vi "GUI_TestStand_Screen1.vi"() -> ()   [LabVIEW 2013]
uses:
  Shared/GUI_Template/GUI_master/tcp_new_data_event.ctl
  Shared/GUI_Template/GUI_master/tcp new data cluster.ctl
  Fire button.ctl
panel:
  in  "RepRate::6":dbl=25.5 caption="Rep\nrate" min=0.0 max=0.0 format="%#.2f"
  out "flow::11":dbl=25.5 caption="PR4000 Flow" min=0.0 max=0.0 format="%_4f"
  out "pressure chart":dbl(graph) caption="Baratron pressure"
  in  "MaxCounts::13":dbl=25.5 caption="Max counts TS-ChromexCam" min=0.0 max=1000.0 format="%_4f"
  out "OK Button 4":bool
  in  "MaxCounts::14":dbl=25.5 caption="Max counts TS-InputNearField" min=0.0 max=1000.0 format="%_4f"
  out "OK Button 3":bool
  in  "MaxCounts::12":dbl=25.5 caption="Max counts TS-Mode1" min=0.0 max=999999999.0 format="%_4f"
  out "OK Button 2":bool
  in  "valve::11":bool caption="Valve"
  in  "pressure::11":dbl=25.5 caption="PR4000 Pressure" min=0.0001 max=30.0 format="%_4f"
  in  "BaratronPressure::9":dbl=25.5 caption="Baratron Pressure" min=0.01 max=10.0 format="%_4f"
  in  "GUIdevice 14":string="TS-InputNearField"
  in  "trigger::14":bool caption="TS-InputNearField"
  in  "trigger::13":bool caption="TS-ChromexCam"
  in  "GUIdevice 13":string="TS-ChromexCam"
  in  "trigger::12":bool caption="TS-Mode1"
  in  "GUIdevice 12":string="TS-Mode1"
  in  "trigger::8":bool caption="TS-Periscope"
  in  "GUIdevice 11":string="TS-PR4000"
  in  "fire::6":string="TS-shotcontrol"
  in  "Fire Button":T1
  in  "Mode::6":bool caption="Mode"
  out "transmission chart":dbl(graph) caption="Transmission [%]"
  in  "EnergyIn::10":dbl=25.5 caption="Pulse energy [uJ]" min=-5.0 max=5.0 format="%_3f"
  in  "EnergyTransmission::10":dbl=-1.0 caption="Transmission [%]" min=0.0001 max=30.0 format="%_3f"
  in  "GUIdevice 10":string="TS-Analysis"
  in  "GUIdevice 9":string="GP1teststand"
  out "OK Button":bool
  in  "MaxCounts::8":dbl=25.5 caption="Max counts TS-Periscope" min=0.01 max=10.0 format="%_4f"
  in  "GUIdevice 8":string="TS-Periscope"
  in  "Trigger.Low Level::7":dbl caption="Level" min=-0.1 max=0.1
  in  "Trigger.Mode::7":T2(ring) caption="Mode"
  in  "delay.Channel_A::4":dbl=40.15 caption="Delay A" min=-0.1 max=0.1 format="%^_4g"
  in  "delay.Channel_D::5":dbl=40.15 caption="Delay D" min=-0.1 max=0.1 format="%_4f"
  in  "delay.Channel_C::5":dbl=40.15 caption="Delay C" min=-0.1 max=0.1 format="%^_6e"
  in  "delay.Channel_B::5":dbl=40.15 caption="Delay B" min=-0.1 max=0.1 format="%_4f"
  in  "delay.Channel_A::5":dbl=40.15 caption="Delay A" min=-0.1 max=0.1 format="%^_6e"
  in  "delay.Channel_D::4":dbl=40.15 caption="Delay D" min=-0.1 max=0.1 format="%_4f"
  in  "delay.Channel_C::4":dbl=40.15 caption="Delay C" min=0.1 max=10.0 format="%_4f"
  in  "delay.Channel_B::4":dbl=40.15 caption="Delay B" min=-0.1 max=0.1 format="%_4f"
  in  "Digitizer Traces":T3 {"offset::7" min=0.0 max=5000.0 format="%_4f"; "verticalrange::7" min=0.0 max=500.0 format="%_4f"}
  in  "position::3":dbl=40.15 caption="Arcus 2 stage \nposition" min=-7.5 max=7.5 format="%_4f"
  in  "position::2":dbl=25.5 caption="Arcus 1 stage" min=-25.0 max=25.0 format="%_4f"
  in  "wangle::1":dbl caption="w" min=0.0 max=50.0 format="%_4f"
  in  "vangle::1":dbl caption="v" min=0.0 max=50.0 format="%_4f"
  in  "uangle::1":dbl=0.5 caption="u" min=0.0 max=50.0 format="%_4f"
  in  "ypos::1":dbl caption="y" min=-7.5 max=7.5 format="%_4f"
  in  "zpos::1":dbl caption="z" min=-12.0 max=12.0 format="%_4f"
  in  "xpos::1":dbl=0.5 caption="x" min=-25.0 max=25.0 format="%_4f"
  in  "GUIdevice 7":string="TS-digitizer-1"
  out "error IO 2":errorcluster
  in  "insert tag":bool=TRUE
  out "tcp data event":T4
  in  "GUIdevice 5":string="TS-dg535-2"
  in  "GUIdevice 4":string="TS-dg535-1"
  in  "GUIdevice 6":string="TS-shotcontrol"
  in  "GUIdevice 3":string="TSArcus2"
  in  "GUIdevice 2":string="TSArcus1"
  in  "GUIdevice 1":string="TS-hexapod"
  in  "stop":bool
  in  "UDP error message":string
  # "TEST STAND CONTROL CENTER"
  # "DIGITIZER"
  # "FOCUS LENS"
  # "SHOT CONTROL"
  # "Trigger"
  # "Camera triggers"
  # "Pressures"
  # "CALCULATIONS"
  # "DG 1"
  # "DG 2"
  # "MODE 1"
  # "HEXAPOD"
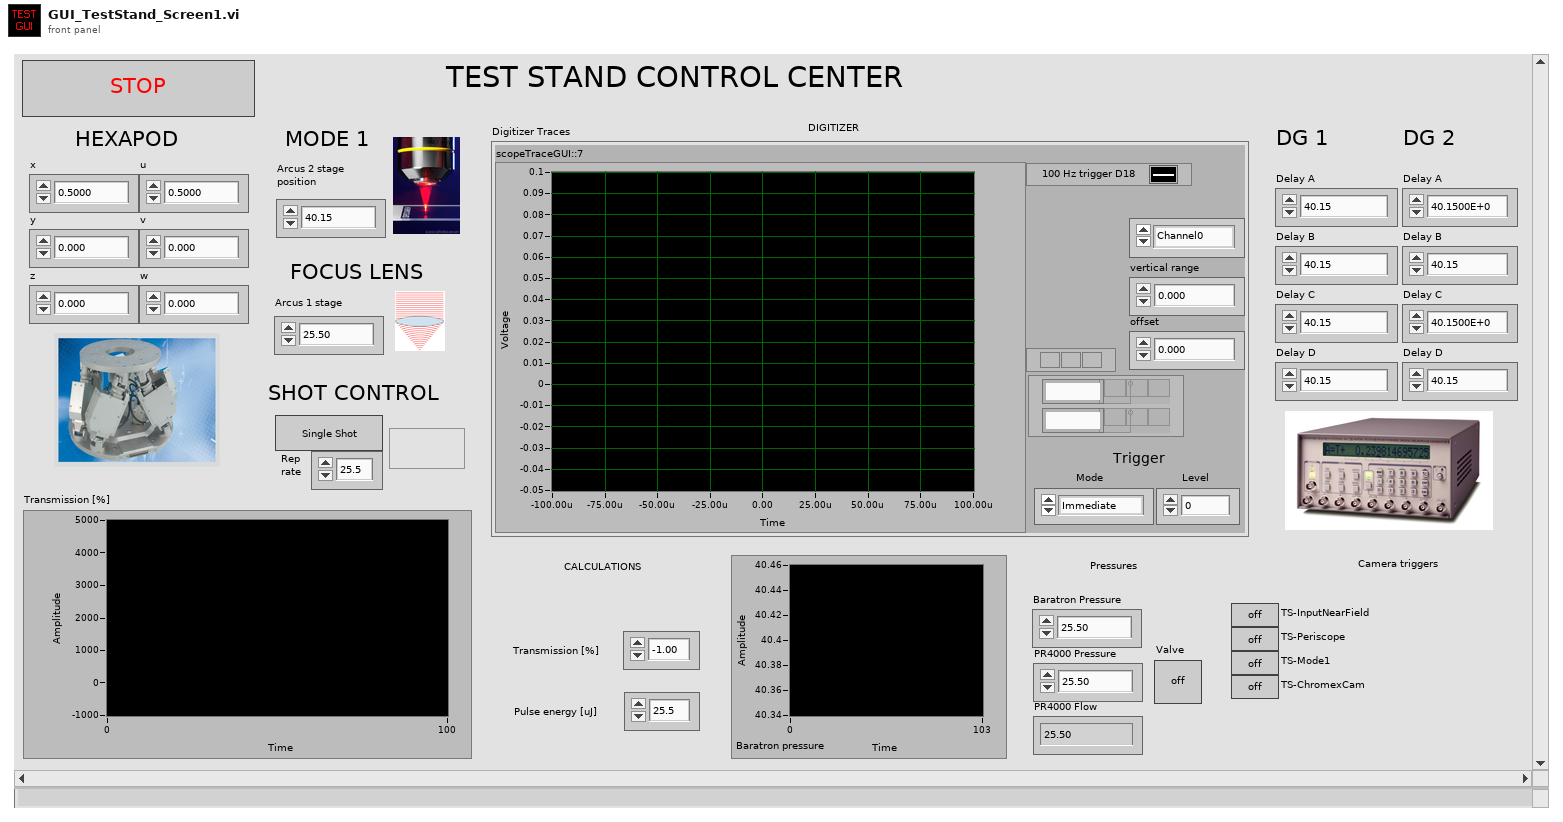
[diagram p1: front panel]
types:
  T1 = typedef "Fire button.ctl" = bool
  T2 = enum16{"Immediate", "Analog Edge", "Analog Window", "Analog Hysteresis", "Video", "Digital Edge"}
  T3 = cluster{"verticalrange::7":dbl, "Channel::7":enum16{"Channel0", "Channel1", "Channel2"}, "scopeTraceGUI::7":waveform(dbl)[], "offset::7":dbl}
  T4 = typedef "tcp_new_data_event.ctl" = refnum<user-event>
  T5 = typedef "tcp new data cluster.ctl" = cluster{"EventEnum":enum16{"new data", "connection status update"}, "Device name":string}
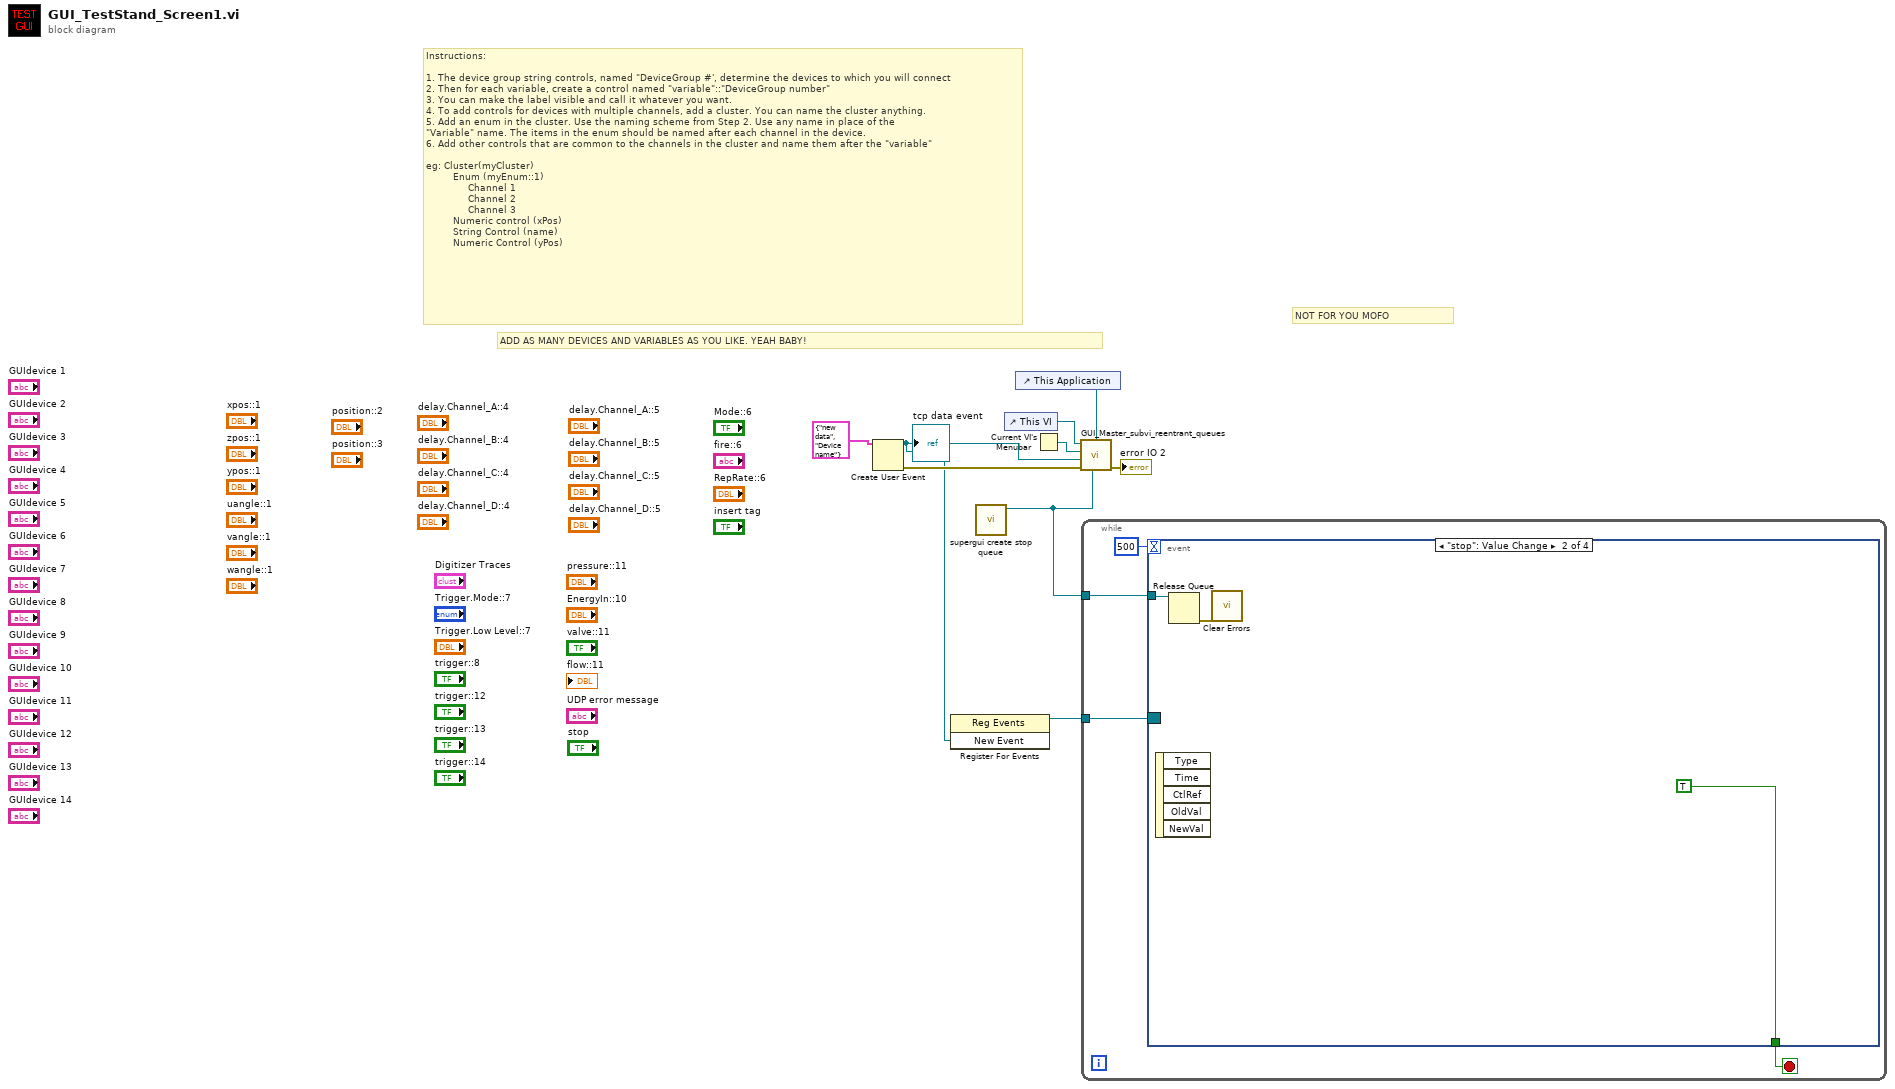
[diagram p0: block diagram]
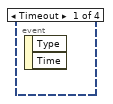
[diagram p2: hidden frame]
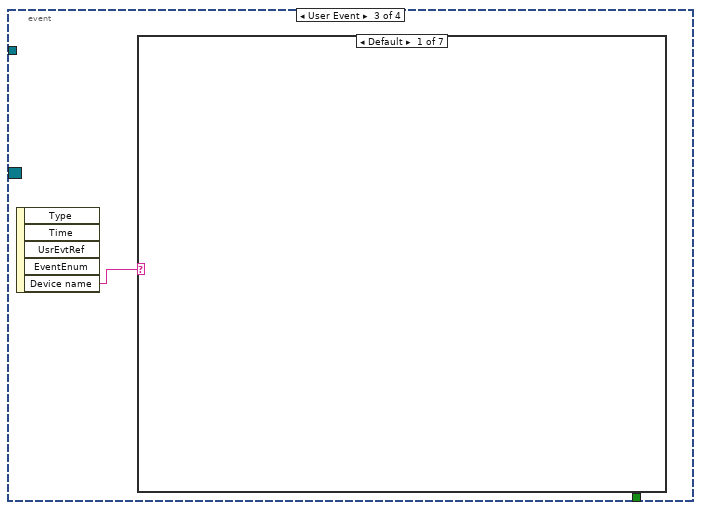
[diagram p3: hidden frame]
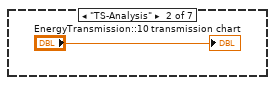
[diagram p4: hidden frame]
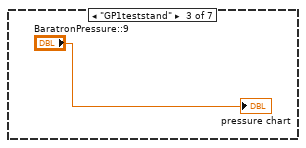
[diagram p5: hidden frame]
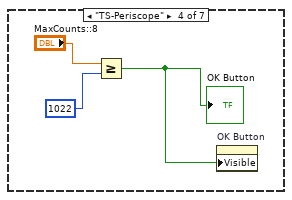
[diagram p6: hidden frame]
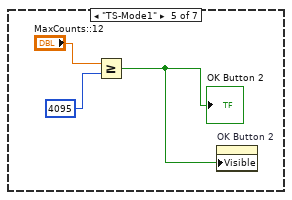
[diagram p7: hidden frame]
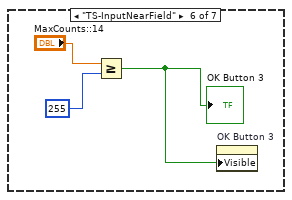
[diagram p8: hidden frame]
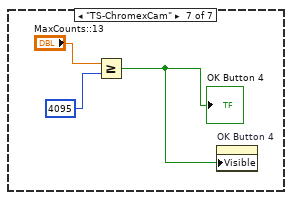
[diagram p9: hidden frame]
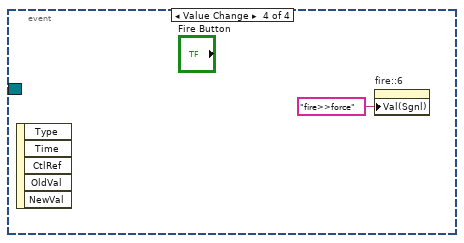
[diagram p10: hidden frame]
diagram:
  # "Instructions:\n\n1. The device group string controls, named \"DeviceGroup #', determine the devices to which you will connect\n2. Then for each variable, create a control named \"variable\"::\"DeviceGroup number\"\n3. You can make the label visible and call it whatever you want.\n4. To add controls for devices with multiple channels, add a cluster. You can name the cluster anything.\n5. Add an enum in the cluster. Use the naming scheme from Step 2. Use any name in place of the \n\"Variable\" name. The items in the enum should be named after each channel in the device. \n6. Add other controls that are common to the channels in the cluster and name them after the \"variable\"\n\neg: Cluster(myCluster)\n         Enum (myEnum::1)\n              Channel 1 \n              Channel 2\n              Channel 3\n         Numeric control (xPos)\n         String Control (name)\n         Numeric Control (yPos)"
  # "ADD AS MANY DEVICES AND VARIABLES AS YOU LIKE. YEAH BABY!"
  # "NOT FOR YOU MOFO"
  n1 = Create User Event(user event datatype=T5 {"EventEnum"=enum."new data", "Device name"="Device name"} ("New Event")) -> (user event=w4:refnum<user-event>, error out=w9:errorcluster)  [unwired: 1 in]
  "tcp data event" <- w4
  n2 = register-events(w4) -> (reference out=w3:refnum<event-registration>)  [unwired: 2 in, 1 out]
  n3 = call "supergui create stop queue.vi"() -> ("STOP Queue out"=w1:refnum<queue>)  [unwired: 11 in]
  n4 = control-ref of="This VI"() -> (w6:refnum<vi>)
  n5 = control-ref of="This Application"() -> (w2:refnum<vi>)
  n6 = Current VI's Menubar() -> (w7:refnum<k9>)
  n7 = call "GUI_Master_subvi_reentrant_queues.vi"("STOP Queue in"=w1, "This Application"=w2, "error in (no error)"=w9, "tcp data event"=w4, "Caller menu reference"=w7, "Caller VI ref"=w6) -> ("error out"=→"error IO 2":errorcluster)  [unwired: 5 in]
  n8 = while {
    tunnel: w3 -> [w13]
    tunnel: w1 -> [w10]
    stop <- w11 stop-if-true
    n9 = event shown="[1] \"stop\": Value Change" {
      selector: w13 -> [_ _ _ _]
      dyn-events: _ -> [_ _ _ _]
      timeout: 500 -> [_ _ _ _]
      tunnel: [_ TRUE _ _] -> w11
      tunnel: w10 -> [_ w15 _ _]
      event Timeout {
        n10 = event-data() -> ()  [unwired: 1 in, 2 out]
      }
      event "stop": Value Change {
        n11 = event-data() -> ()  [unwired: 1 in, 5 out]
        n12 = Release Queue(queue=w15) -> (error out=w14:errorcluster)  [unwired: 2 in, 2 out]
        n13 = call <vilib>:"Clear Errors.vi"("error in (no error)"=w14) -> ()  [unwired: 6 in, 1 out]
      }
      event User Event {
        n14 = event-data() -> ("Device name"=w17:string)  [unwired: 1 in, 4 out]
        n15 = case shown="Default" w17 {
          frame Default {
          }
          frame "TS-Analysis" {
            "transmission chart" <- "EnergyTransmission::10"
          }
          frame "GP1teststand" {
            "pressure chart" <- "BaratronPressure::9"
          }
          frame "TS-Periscope" {
            n16 = Greater Or Equal?(x="MaxCounts::8", y=1022) -> (x >= y?=w20:bool)
            "OK Button" <- w20
            n17 = property on="OK Button" class="Bool"("Visible"=w20) -> ()  [unwired: 2 in, 2 out]
          }
          frame "TS-Mode1" {
            n18 = Greater Or Equal?(x="MaxCounts::12", y=4095) -> (x >= y?=w23:bool)
            "OK Button 2" <- w23
            n19 = property on="OK Button 2" class="Bool"("Visible"=w23) -> ()  [unwired: 2 in, 2 out]
          }
          frame "TS-InputNearField" {
            n20 = Greater Or Equal?(x="MaxCounts::14", y=255) -> (x >= y?=w26:bool)
            "OK Button 3" <- w26
            n21 = property on="OK Button 3" class="Bool"("Visible"=w26) -> ()  [unwired: 2 in, 2 out]
          }
          frame "TS-ChromexCam" {
            n22 = Greater Or Equal?(x="MaxCounts::13", y=4095) -> (x >= y?=w29:bool)
            "OK Button 4" <- w29
            n23 = property on="OK Button 4" class="Bool"("Visible"=w29) -> ()  [unwired: 2 in, 2 out]
          }
        }
      }
      event Value Change {
        n24 = event-data() -> ()  [unwired: 1 in, 5 out]
        n25 = property on="fire::6" class="Str"("Val(Sgnl)"="fire>>force" ("Value (Signaling)")) -> ()  [unwired: 2 in, 2 out]
      }
    }
  }
